vi "Store Last Command (SubVI).vi"(7 "Command":T2, 8 "error in":errorcluster, 11 "Storage Command":T1=enum."Operator") -> (0 "error out":errorcluster, 3 "Last Command":T1)   [LabVIEW 2012]
doc: "FGV to used to store commands, used typically to store the last command. This is as certain command have different behaviour depending upon the last command issued."
uses:
  Controls/Command Enum.ctl
  Controls/Storing Commands.ctl
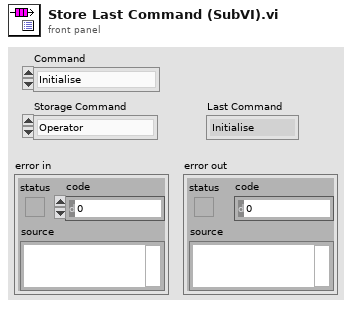
[diagram p1: front panel]
types:
  T1 = typedef "Command Enum.ctl" = enum16{"Initialise", "Data Entry", "Decimal Point", "Operator", "Calculation", "Backspace", "Clear Line", "Clear All", "Close"}
  T2 = typedef "Storing Commands.ctl" = enum16{"Initialise", "GET", "SET"}
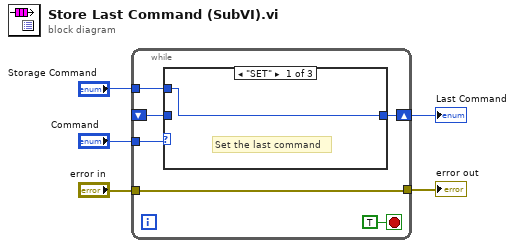
[diagram p0: block diagram]
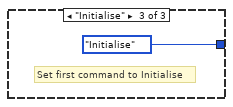
[diagram p3: hidden frame]
diagram:
  n1 = while {
    tunnel: "error in" -> [w11]
    tunnel: [w11] -> w5
    tunnel: "Command" -> [w9]
    shift-right: [w8] -> w2
    shift-left: _ -> [w7]
    tunnel: "Storage Command" -> [w6]
    stop <- TRUE stop-if-true
    n2 = case shown="\"SET\"" w9 {
      tunnel: [w12 w13 Command_Enum."Initialise" ("Command")] -> w8
      tunnel: w7 -> [_ w13 _]
      tunnel: w6 -> [w12 _ _]
      frame "SET" {
        # "Set the last command"
      }
      frame "GET" {
        # "Return the last stored command"
      }
      frame "Initialise" {
        # "Set first command to Initialise"
      }
    }
  }
  "error out" <- w5
  "Last Command" <- w2
